vi "bbauv_acoustic.vi"() -> ()   [LabVIEW 2012]
doc: "This VI will initialize the FPGA VI and read a user-defined number of samples from a DMA FIFO. When the data acquisition is complete this VI will read status information from the FPGA VI.\n\nFollow these instructions to run the VI.\n\n1. Select your RIO device from the dropdown.\n2. Set the sample period, number of samples to acquire per channel, and DMA block read size. \n\nNote: the block read size should be set to balance load on the host processor and the update rate of the user interface. A small block read size will update the user interface more often but will result in a higher load on the host processor."
uses:
  <vilib>/userdefined/High Color/nirio_resource_hc.ctl
  <vilib>/FPGAPlugInAG/sbRIO-9612/niLvFpga_Open_sbRIO-9612.vi
  <vilib>/rvi/interface/common/dynamic/niFpgaDynamicAddResources.vi
  <vilib>/Utility/error.llb/Error Cluster From Error Code.vi
  <vilib>/FPGAPlugInAG/Dynamic/niLvFpga_Run_Dynamic.vi
  <vilib>/rvi/errors/niLvFpgaAdjustHostInterfaceError.vi
  <vilib>/RVI Host/nirviSupport.llb/nirviErrorClusterFromErrorCode.vi
  <vilib>/FPGAPlugInAG/Dynamic/niLvFpga_Close_Dynamic.vi
  <vilib>/express/express analysis/Spectral/Block/exnSpectralBlock spectral measurements peak poly.vi
  <vilib>/express/express analysis/Spectral/Block/exnSpectralBlock spectral measurements peak DDT.vi
  <vilib>/rvi/interface/nirviOpenFPGA/nirviOpenFPGA.xnode
  FPGA Bitfiles/bbauvFPGA_FPGATarget2_NI9223User-Contr_AXBjtBmtN8Y.lvbitx
  NI 9223 User-Controlled IO Sampling (FPGA).vi
  <vilib>/rvi/interface/nirviMethod/nirviMethod.xnode
  <vilib>/rvi/interface/nirviReadWriteControl/nirviReadWriteControl.xnode
  <vilib>/rvi/interface/nirviCloseFPGA/nirviCloseFPGA.xnode
  <vilib>/express/express analysis/Spectral/XNode/ExpressSpectralMeasurementsBlockNode.xnode
  <vilib>/rvi/errors/niLvFpgaMergeErrorWithErrorCode.vi
  <vilib>/rvi/interface/Simulation/niFpgaSimulationCallBeginRW.vi
  <vilib>/FPGAPlugInAG/Dynamic/niLvFpga_ReadFifo_Dynamic.vi
  <vilib>/rvi/interface/nirviMethod/StockFPGA_InlinedMethodWaitForSingleIRQ.vi
  <vilib>/FPGAPlugInAG/Dynamic/niLvFpga_WaitOnIrq_Dynamic.vi
  <vilib>/FPGAPlugInAG/Dynamic/niLvFpga_AcknowledgeIrq_Dynamic.vi
  NiFpgaLv.dll
  <vilib>/FPGAPlugInAG/Dynamic/niLvFpga_ConfigureFifo_Dynamic.vi
  <vilib>/FPGAPlugInAG/Dynamic/niLvFpga_StartFifo_Dynamic.vi
panel:
  out "Yaw Chart":dbl(graph)
  in  "Operating Mode":T1(ring)=enum."Analyze Real-time"
  in  "Filename":path=path "D:/Record Signal/sig 1.lvm"
  out "dt1":dbl
  out "dt2":dbl
  out "dt3":dbl
  out "Index 0":dbl
  out "Index 1":dbl
  out "Index 2":dbl
  out "Index 3":dbl
  out "ratio":dbl
  out "ratio 2":dbl
  out "ratio 3":dbl
  out "ratio 4":dbl
  out "amplitude":dbl
  out "amplitude 2":dbl
  out "amplitude 3":dbl
  out "amplitude 4":dbl
  out "ROS  Error":bool
  in  "Manual depth":dbl=4.3
  in  "Mode":T2(ring)=enum."Use Far Field"
  out "x":dbl format="%#_6f"
  out "y":dbl format="%#_6f"
  out "z":dbl
  out "yaw":dbl
  out "pitch":dbl
  out "Selected Index":i32
  in  "LPF Cut-Off":dbl=40000.0 caption="Lower Cut-Off"
  out "Ratio at Index (%)":dbl
  in  "Portion Duration":i32=200
  in  "peak min":dbl=0.1
  in  "Threshold":dbl=0.1
  out "Freq Domain":dynamicdata(graph)
  out "#element acquired":u32(graph)
  in  "Sampling Duration (us)":u32=2050000
  in  "RIO Device":T3="rio://192.168.0.150/RIO0"
  out "Timed Out":bool
  out "Sample Gated":bool
  out "Overwrite":bool
  in  "Acquisition Stop":bool
  out "Portion":dynamicdata(graph)
  out "Orignal Signal":dynamicdata(graph)
  # "Peak Finding"
  # "Triangulation Result"
  # "Operating Control"
  # "TDOA (us)"
  # "Signal Analysis Control"
  # "Signal Acquisition Control"
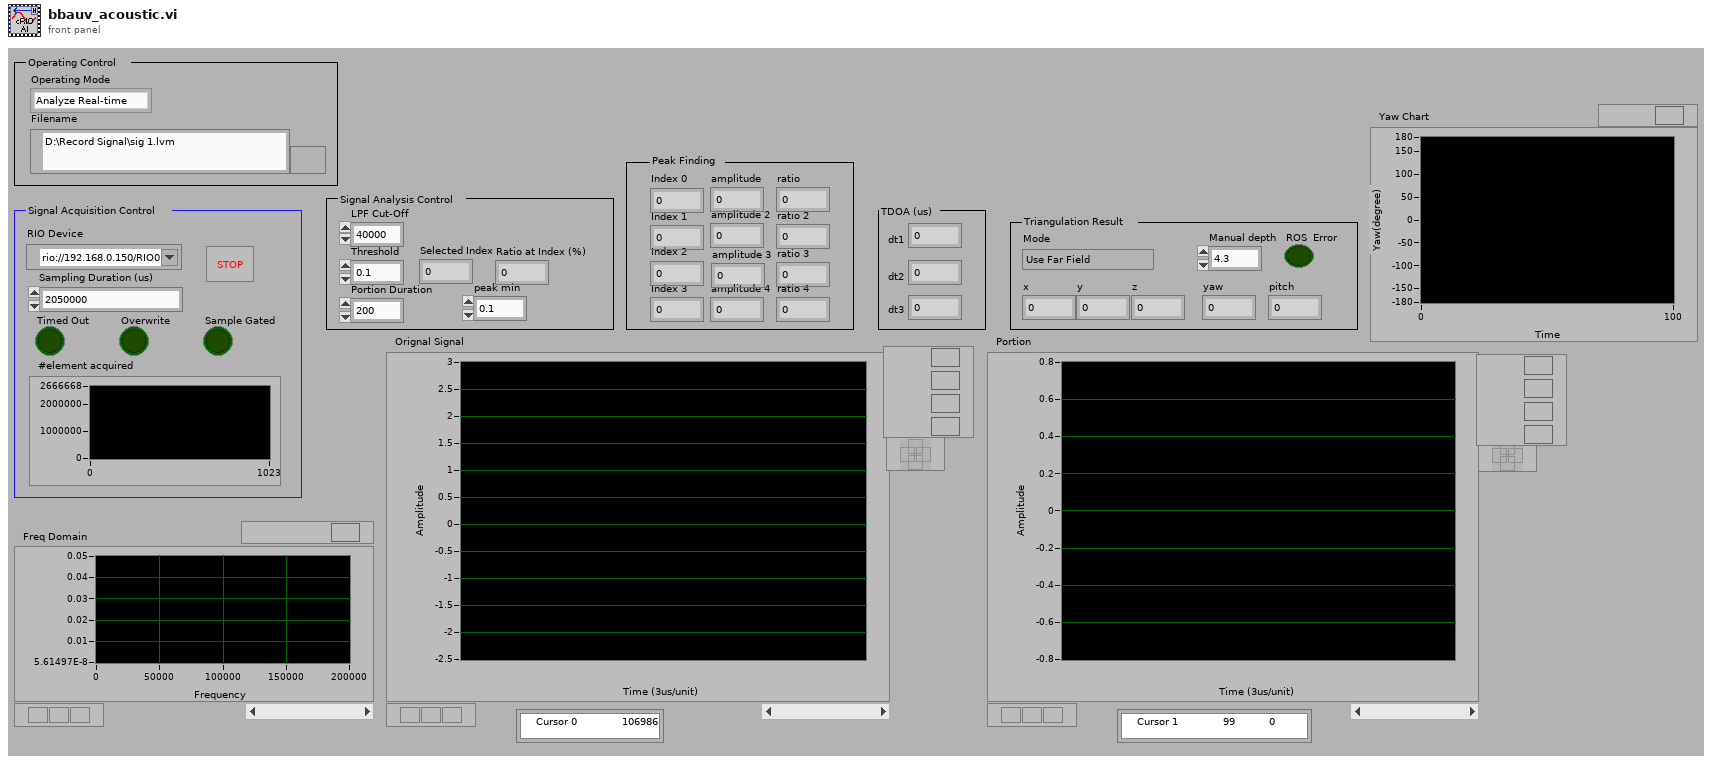
[diagram p1: front panel]
types:
  T1 = enum16{"Analyze From File", "Record Data", "Analyze Real-time"}
  T2 = enum16{"Use Near Field", "Use Far Field", "Send to ROS", "Far Field with 3 hydrophones"}
  T3 = typedef "nirio_resource_hc.ctl" = tag
  T4 = cluster{"averaging mode":u16, "weighting mode":u16, "number of averages":u32}
  T5 = cluster{"dB On (F)":bool, "unwrap phase (F)":bool, "convert to degree (F)":bool}
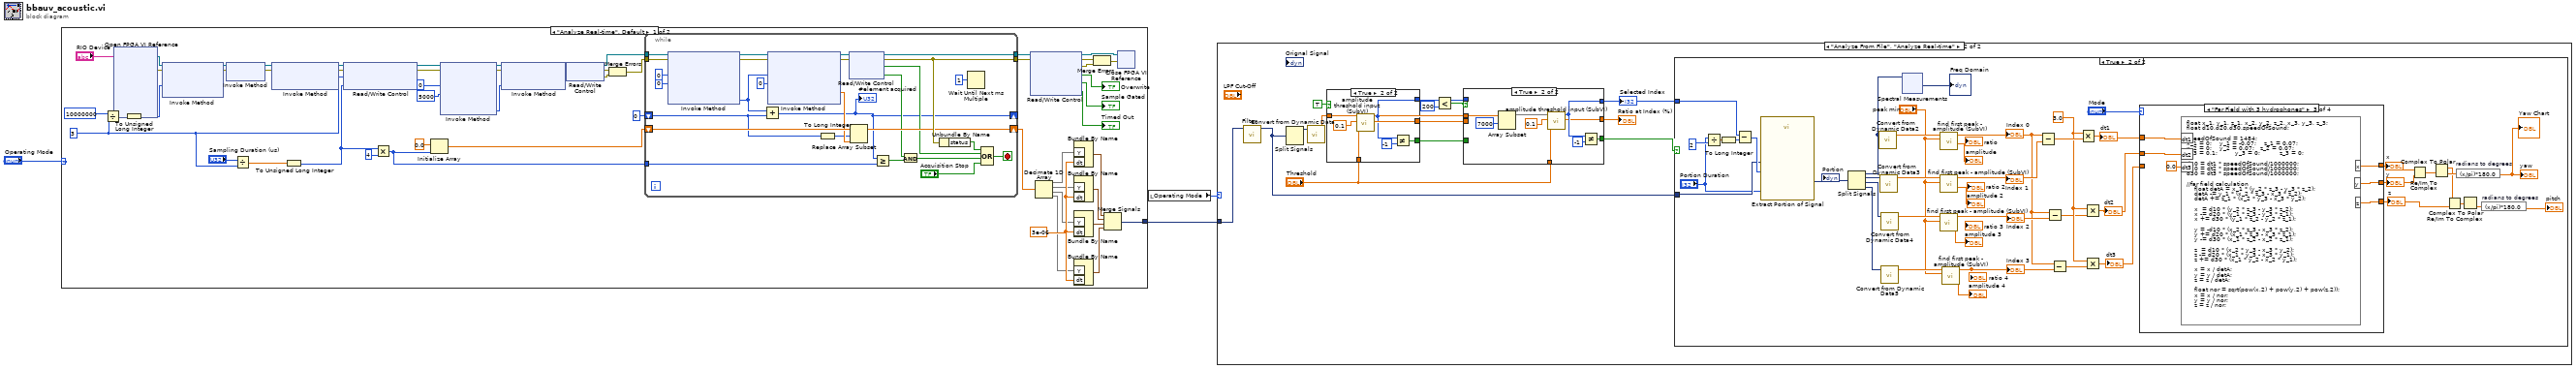
[diagram p0: block diagram]
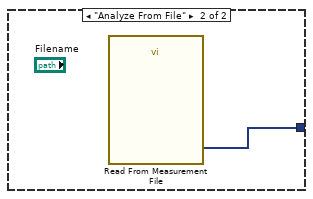
[diagram p2: hidden frame]
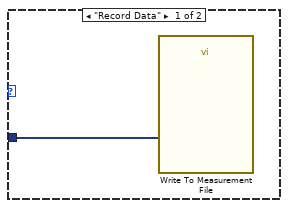
[diagram p3: hidden frame]
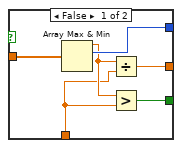
[diagram p5: hidden frame]
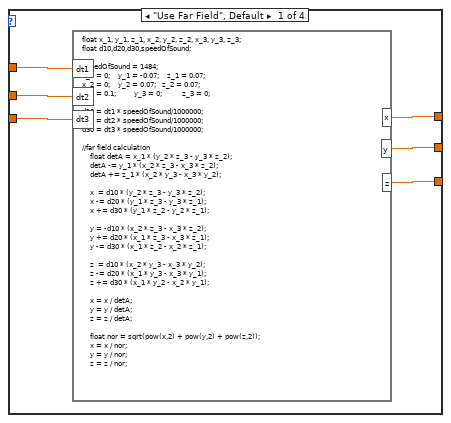
[diagram p7: hidden frame]
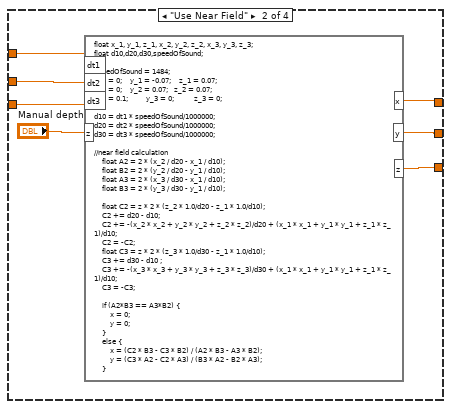
[diagram p8: hidden frame]
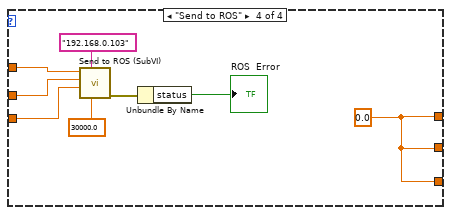
[diagram p9: hidden frame]
diagram:
  n1 = case shown="\"Analyze Real-time\", Default" "Operating Mode" {
    tunnel: [w8 w85] -> w3
    frame "Analyze Real-time", Default {
      w7 = u32 3 ("Sample Period (uSec)")
      w17 = 3e-06 ("dt")
      n2 = Divide(x=u32 10000000, y=w7) -> (x/y=w51:dbl)
      n3 = xnode "Open FPGA VI Reference"("resource name"="RIO Device") -> ("FPGA VI Reference Out"=w54:refnum<k20>, "error out"=w53:errorcluster)  [unwired: 1 in]
      n4 = To Unsigned Long Integer(number=w51) -> (unsigned 32bit integer=w52:u32)
      n5 = xnode "Invoke Method"("FPGA VI Reference In"=w54, "error in"=w53, "Requested Depth"=w52) -> ("FPGA VI Reference Out"=w56:refnum<k20>, "error out"=w55:errorcluster)  [unwired: 1 out]
      n6 = xnode "Invoke Method"("FPGA VI Reference In"=w56, "error in"=w55) -> ("FPGA VI Reference Out"=w45:refnum<k20>, "error out"=w44:errorcluster)
      n7 = Divide(x="Sampling Duration (us)", y=w7) -> (x/y=w5:dbl)
      n8 = xnode "Invoke Method"("FPGA VI Reference In"=w45, "error in"=w44) -> ("FPGA VI Reference Out"=w21:refnum<k20>, "error out"=w20:errorcluster)  [unwired: 1 in]
      n9 = To Unsigned Long Integer(number=w5) -> (unsigned 32bit integer=w4:u32)
      n10 = xnode "Read/Write Control"("FPGA VI Reference In"=w21, "error in"=w20, "Sample Period (uSec)"=w7, "Number of Samples"=w4) -> ("FPGA VI Reference Out"=w35:refnum<k20>, "error out"=w34:errorcluster)
      n11 = Multiply(x=w4, y=u32 4) -> (x*y=w48:u32)
      n12 = Initialize Array(sgl 0.0, w48) -> (w24:sgl[])
      n13 = xnode "Invoke Method"("FPGA VI Reference In"=w35, "error in"=w34, "IRQ Number(s)"=0, "Timeout (ms)"=5000) -> ("FPGA VI Reference Out"=w32:refnum<k20>, "error out"=w33:errorcluster, "IRQ(s) Asserted"=w29:i32)  [unwired: 1 out]
      n14 = xnode "Invoke Method"("FPGA VI Reference In"=w32, "error in"=w33, "IRQ Number(s)"=w29) -> ("FPGA VI Reference Out"=w31:refnum<k20>, "error out"=w30:errorcluster)
      n15 = xnode "Read/Write Control"("FPGA VI Reference In"=w31, "error in"=w30) -> ("FPGA VI Reference Out"=w23:refnum<k20>, "error out"=w37:errorcluster, "Error Out"=w36:errorcluster)
      n16 = Merge Errors(w37, w36) -> (w22:errorcluster)
      n17 = while {
        tunnel: w23 -> [w71]
        tunnel: w22 -> [w70]
        tunnel: [w79] -> w43
        tunnel: [w78] -> w42
        shift-right: [w58] -> _
        shift-left: u32 0 -> [w72]
        tunnel: w48 -> [w63]
        shift-right: [w74] -> w13
        shift-left: w24 -> [w80]
        stop <- w81 stop-if-true
        n18 = xnode "Invoke Method"("FPGA VI Reference In"=w71, "error in"=w70, "Number of Elements"=u32 0, "Timeout (ms)"=0) -> ("FPGA VI Reference Out"=w69:refnum<k20>, "error out"=w68:errorcluster, "Elements Remaining"=w59:u32)  [unwired: 1 out]
        n19 = Add(x=w59, y=w72) -> (x+y=w58:u32)
        "#element acquired" <- w58
        n20 = xnode "Invoke Method"("FPGA VI Reference In"=w69, "error in"=w68, "Number of Elements"=w59, "Timeout (ms)"=0) -> ("FPGA VI Reference Out"=w84:refnum<k20>, "error out"=w83:errorcluster, "Data"=w75:sgl[])  [unwired: 1 out]
        n21 = To Long Integer(number=w72) -> (32bit integer=w73:i32)
        n22 = xnode "Read/Write Control"("FPGA VI Reference In"=w84, "error in"=w83) -> ("FPGA VI Reference Out"=w79:refnum<k20>, "error out"=w78:errorcluster, "Error"=w60:bool, "Stopped"=w62:bool)
        n23 = Replace Array Subset(array=w80, new element=w75, index=w73) -> (w74:sgl[])
        n24 = Greater Or Equal?(x=w58, y=w63) -> (x >= y?=w64:bool)
        n25 = And(x=w62, y=w64) -> (x .and. y?=w61:bool)
        n26 = Unbundle By Name(w78) -> ("status"=w65:bool)
        n27 = Wait Until Next ms Multiple(millisecond multiple=u32 1) -> ()  [unwired: 1 out]
        n28 = Compound Arithmetic op=OR(w65, w60, w61, "Acquisition Stop") -> (w81:bool)
      }
      n29 = xnode "Read/Write Control"("FPGA VI Reference In"=w43, "error in"=w42) -> ("FPGA VI Reference Out"=w47:refnum<k20>, "error out"=w38:errorcluster, "Error Out"=w39:errorcluster, "Overwrite"=→"Overwrite":bool, "Sample Gated"=→"Sample Gated":bool, "Timed Out"=→"Timed Out":bool)
      n30 = Decimate 1D Array(w13) -> (w12:sgl[], w11:sgl[], w9:sgl[], w10:sgl[])
      n31 = Bundle By Name("Y"=w12, "dt"=w17) -> (w14:waveform(sgl))  [unwired: 1 in]
      n32 = Bundle By Name("Y"=w11, "dt"=w17) -> (w15:waveform(sgl))  [unwired: 1 in]
      n33 = Bundle By Name("Y"=w9, "dt"=w17) -> (w16:waveform(sgl))  [unwired: 1 in]
      n34 = Bundle By Name("Y"=w10, "dt"=w17) -> (w18:waveform(sgl))  [unwired: 1 in]
      n35 = Merge Errors(w38, w39) -> (w46:errorcluster)
      n36 = Merge Signals(w14, w15, w16, w18) -> (w8:dynamicdata)
      n37 = xnode "Close FPGA VI Reference"("FPGA VI Reference In"=w47, "error in"=w46) -> ()  [unwired: 1 out]
    }
    frame "Analyze From File" {
      n38 = call "Read From Measurement File"() -> ("Signals"=w85:dynamicdata)  [unwired: 6 in, 5 out]
    }
  }
  n39 = local read "Operating Mode"() -> (w2:T1)
  n40 = case shown="\"Analyze From File\", \"Analyze Real-time\"" w2 {
    tunnel: w3 -> [w86 w88]
    frame "Record Data" {
      n41 = call "Write To Measurement File"("Signals"=w86) -> ()  [unwired: 16 in, 3 out]
    }
    frame "Analyze From File", "Analyze Real-time" {
      n42 = call "Filter"("Signal"=w88) -> ("Filtered Signal"=w89:dynamicdata)  [unwired: 9 in, 1 out]
      n43 = Split Signals(w89) -> (w87:dynamicdata)  [unwired: 4 in, 3 out]
      n44 = call "Convert from Dynamic Data"("Dynamic Data Type"=w87) -> ("Array"=w95:dbl[])  [unwired: 3 in]
      n45 = case shown="True" TRUE {
        tunnel: w95 -> [w118 w125]
        tunnel: [w115 w122] -> w96
        tunnel: [w116 w121] -> w91
        tunnel: [w117 w120] -> w99
        tunnel: "Threshold" -> [w113 w119]
        frame False {
          n46 = Array Max & Min(array=w118) -> (max value=w114:dbl, max index (indices)=w116:i32)  [unwired: 2 out]
          n47 = Divide(x=w114, y=w113) -> (x/y=w115:dbl)
          n48 = Greater?(x=w114, y=w113) -> (0:w117:bool)
        }
        frame True {
          n49 = call "amplitude threshold input (SubVI).vi"("threshold"=w119, "%max amplitude"=0.1, "Array"=w125) -> ("actual ratio (%)"=w122:dbl, "Index"=w121:i32)  [unwired: 7 in]
          n50 = Not Equal?(x=w121, y=-1) -> (x != y?=w120:bool)
        }
      }
      n51 = Less?(x=w91, y=200) -> (x < y?=w97:bool)
      n52 = case shown="True" w97 {
        tunnel: w99 -> [w103 _]
        tunnel: w96 -> [w101 _]
        tunnel: w95 -> [_ w112]
        tunnel: "Threshold" -> [_ w107]
        tunnel: [w103 w106] -> w93
        tunnel: [w102 w105] -> w90
        tunnel: [w101 w104] -> w92
        tunnel: w91 -> [w102 _]
        frame False {
        }
        frame True {
          n53 = Array Subset(array=w112, index=7000) -> (w108:dbl[])  [unwired: 1 in]
          n54 = call "amplitude threshold input (SubVI).vi"("threshold"=w107, "%max amplitude"=0.1, "Array"=w108) -> ("actual ratio (%)"=w104:dbl, "Index"=w105:i32)  [unwired: 7 in]
          n55 = Not Equal?(x=w105, y=-1) -> (x != y?=w106:bool)
        }
      }
      "Ratio at Index (%)" <- w92
      "Selected Index" <- w90
      n56 = case shown="True" w93 {
        tunnel: w89 -> [_ w166]
        tunnel: w90 -> [_ w132]
        frame False {
        }
        frame True {
          w162 = 3.0 ("x")
          n57 = Divide(x="Portion Duration", y=2) -> (x/y=w136:dbl)
          n58 = To Long Integer(number=w136) -> (32bit integer=w135:i32)
          n59 = Subtract(x=w132, y=w135) -> (x-y=w169:i32)
          n60 = call "Extract Portion of Signal"("Samples"="Portion Duration", "Begin Sample"=w169, "Signals"=w166) -> ("Section"=w165:dynamicdata)  [unwired: 7 in, 1 out]
          "Portion" <- w165
          n61 = Split Signals(w165) -> (w126:dynamicdata, w168:dynamicdata, w167:dynamicdata, w164:dynamicdata)  [unwired: 4 in]
          n62 = call "Convert from Dynamic Data2"("Dynamic Data Type"=w126) -> ("Array"=w157:dbl[])  [unwired: 3 in]
          n63 = call "Convert from Dynamic Data3"("Dynamic Data Type"=w168) -> ("Array"=w156:dbl[])  [unwired: 3 in]
          n64 = call "Convert from Dynamic Data4"("Dynamic Data Type"=w167) -> ("Array"=w155:dbl[])  [unwired: 3 in]
          n65 = call "Convert from Dynamic Data5"("Dynamic Data Type"=w164) -> ("Array"=w154:dbl[])  [unwired: 3 in]
          n66 = xnode "Spectral Measurements"("Signals"=w126) -> ("FFT - (Peak)"=→"Freq Domain":dynamicdata)  [unwired: 1 in, 2 out]
          n67 = call "find first peak - amplitude (SubVI).vi"("min peak amplitude"="peak min", "Array"=w155) -> ("amplitude"=→"amplitude 3":dbl, "Index"=w152:dbl)  [unwired: 6 in, 1 out]
          "Index 2" <- w152
          n68 = call "find first peak - amplitude (SubVI).vi"("min peak amplitude"="peak min", "Array"=w157) -> ("amplitude"=→"amplitude":dbl, "Index"=w151:dbl)  [unwired: 6 in, 1 out]
          "Index 0" <- w151
          n69 = call "find first peak - amplitude (SubVI).vi"("min peak amplitude"="peak min", "Array"=w156) -> ("amplitude"=→"amplitude 2":dbl, "Index"=w153:dbl)  [unwired: 6 in, 1 out]
          "Index 1" <- w153
          n70 = call "find first peak - amplitude (SubVI).vi"("min peak amplitude"="peak min", "Array"=w154) -> ("amplitude"=→"amplitude 4":dbl, "Index"=w150:dbl)  [unwired: 6 in, 1 out]
          "Index 3" <- w150
          n71 = Subtract(x=w151, y=w153) -> (x-y=w163:dbl)
          n72 = Subtract(x=w151, y=w152) -> (x-y=w161:dbl)
          n73 = Subtract(x=w151, y=w150) -> (x-y=w160:dbl)
          n74 = Multiply(x=w162, y=w163) -> (x*y=w139:dbl)
          "dt1" <- w139
          n75 = Multiply(x=w162, y=w161) -> (x*y=w159:dbl)
          "dt2" <- w159
          n76 = Multiply(x=w162, y=w160) -> (x*y=w138:dbl)
          "dt3" <- w138
          n77 = case shown="\"Far Field with 3 hydrophones\"" "Mode" {
            tunnel: w139 -> [w185 w192 w198 w205]
            tunnel: w159 -> [w184 w191 w197 w204]
            tunnel: [w183 w190 w195 w202] -> w146
            tunnel: [w182 w189 w194 w202] -> w145
            tunnel: [w181 w188 w193 w202] -> w144
            tunnel: w138 -> [w180 w186 _ w201]
            frame "Use Far Field", Default {
              n78 = formula code="float x_1, y_1, z_1, x_2, y_2, z_2, x_3, y_3, z_3;\nfloat d10,d20,d30,speedOfSound;\n\nspeedOfSound = 1484;\nx_1 = 0;    y_1 = -0.07;    z_1 = 0.07;\nx_2 = 0;    y_2 = 0.07;   z_2 = 0.07;\nx_3 = 0.1;         y_3 = 0;          z_3 = 0;\n\nd10 = dt1 * speedOfSound/1000000;\nd20 = dt2 * speedOfSound/1000000;\nd30 = dt3 * speedOfSound/1000000;\n\n//far field calculation\n    float detA = x_1 * (y_2 * z_3 - y_3 * z_2);\n    detA -= y_1 * (x_2 * z_3 - x_3 * z_2);\n    detA += z_1 * (x_2 * y_3 - x_3 * y_2);\n\n    x  = d10 * (y_2 * z_3 - y_3 * z_2);\n    x -= d20 * (y_1 * z_3 - y_3 * z_1);\n    x += d30 * (y_1 * z_2 - y_2 * z_1);\n\n    y = -d10 * (x_2 * z_3 - x_3 * z_2);\n    y += d20 * (x_1 * z_3 - x_3 * z_1);\n    y -= d30 * (x_1 * z_2 - x_2 * z_1);\n\n    z  = d10 * (x_2 * y_3 - x_3 * y_2);\n    z -= d20 * (x_1 * y_3 - x_3 * y_1);\n    z += d30 * (x_1 * y_2 - x_2 * y_1);\n\n    x = x / detA;\n    y = y / detA;\n    z = z / detA;\n\n    float nor = sqrt(pow(x,2) + pow(y,2) + pow(z,2));\n    x = x / nor;\n    y = y / nor;\n    z = z / nor;"("dt1"=w185, "dt2"=w184, "dt3"=w180) -> ("x"=w183:dbl, "y"=w182:dbl, "z"=w181:dbl)
            }
            frame "Use Near Field" {
              n79 = formula code="float x_1, y_1, z_1, x_2, y_2, z_2, x_3, y_3, z_3;\nfloat d10,d20,d30,speedOfSound;\n\nspeedOfSound = 1484;\nx_1 = 0;    y_1 = -0.07;    z_1 = 0.07;\nx_2 = 0;    y_2 = 0.07;   z_2 = 0.07;\nx_3 = 0.1;         y_3 = 0;          z_3 = 0;\n\nd10 = dt1 * speedOfSound/1000000;\nd20 = dt2 * speedOfSound/1000000;\nd30 = dt3 * speedOfSound/1000000;\n\n//near field calculation\n    float A2 = 2 * (x_2 / d20 - x_1 / d10);\n    float B2 = 2 * (y_2 / d20 - y_1 / d10);\n    float A3 = 2 * (x_3 / d30 - x_1 / d10);\n    float B3 = 2 * (y_3 / d30 - y_1 / d10);\n    \n    float C2 = z * 2 * (z_2 * 1.0/d20 - z_1 * 1.0/d10);\n    C2 += d20 - d10;\n    C2 += -(x_2 * x_2 + y_2 * y_2 + z_2 * z_2)/d20 + (x_1 * x_1 + y_1 * y_1 + z_1 * z_1)/d10;\n    C2 = -C2;\n    float C3 = z * 2 * (z_3 * 1.0/d30 - z_1 * 1.0/d10);\n    C3 += d30 - d10 ;\n    C3 += -(x_3 * x_3 + y_3 * y_3 + z_3 * z_3)/d30 + (x_1 * x_1 + y_1 * y_1 + z_1 * z_1)/d10;\n    C3 = -C3;\n\n    if (A2*B3 == A3*B2) {\n        x = 0;\n        y = 0;\n    }\n    else {\n        x = (C2 * B3 - C3 * B2) / (A2 * B3 - A3 * B2);\n        y = (C3 * A2 - C2 * A3) / (B3 * A2 - B2 * A3);\n    }"("dt1"=w192, "dt2"=w191, "dt3"=w186, "z"="Manual depth") -> ("x"=w190:dbl, "y"=w189:dbl, "z"=w188:dbl)
            }
            frame "Far Field with 3 hydrophones" {
              n80 = formula code="float x_1, y_1, z_1, x_2, y_2, z_2, x_3, y_3, z_3;\nfloat d10,d20,d30,speedOfSound;\n\nspeedOfSound = 1484;\nx_1 = 0;    y_1 = -0.07;    z_1 = 0.07;\nx_2 = 0;    y_2 = 0.07;   z_2 = 0.07;\nx_3 = 0.1;         y_3 = 0;          z_3 = 0;\n\nd10 = dt1 * speedOfSound/1000000;\nd20 = dt2 * speedOfSound/1000000;\nd30 = dt3 * speedOfSound/1000000;\n\n//far field calculation\n    float detA = x_1 * (y_2 * z_3 - y_3 * z_2);\n    detA -= y_1 * (x_2 * z_3 - x_3 * z_2);\n    detA += z_1 * (x_2 * y_3 - x_3 * y_2);\n\n    x  = d10 * (y_2 * z_3 - y_3 * z_2);\n    x -= d20 * (y_1 * z_3 - y_3 * z_1);\n    x += d30 * (y_1 * z_2 - y_2 * z_1);\n\n    y = -d10 * (x_2 * z_3 - x_3 * z_2);\n    y += d20 * (x_1 * z_3 - x_3 * z_1);\n    y -= d30 * (x_1 * z_2 - x_2 * z_1);\n\n    z  = d10 * (x_2 * y_3 - x_3 * y_2);\n    z -= d20 * (x_1 * y_3 - x_3 * y_1);\n    z += d30 * (x_1 * y_2 - x_2 * y_1);\n\n    x = x / detA;\n    y = y / detA;\n    z = z / detA;\n\n    float nor = sqrt(pow(x,2) + pow(y,2) + pow(z,2));\n    x = x / nor;\n    y = y / nor;\n    z = z / nor;"("dt1"=w198, "dt2"=w197, "dt3"=0.0 ("input variable")) -> ("x"=w195:dbl, "y"=w194:dbl, "z"=w193:dbl)
            }
            frame "Send to ROS" {
              w202 = 0.0 ("x")
              n81 = call "Send to ROS (SubVI).vi"("frequency"=30000.0, "ROS IP"="192.168.0.103", "dt 3"=w201, "dt2"=w204, "dt 1"=w205) -> ("error out"=w200:errorcluster)  [unwired: 6 in]
              n82 = Unbundle By Name(w200) -> ("status"=→"ROS  Error":bool)
            }
          }
          "x" <- w146
          "y" <- w145
          "z" <- w144
          n83 = Re/Im To Complex(1:w145, 2:w146) -> (0:w148:cdb)
          n84 = Complex To Polar(r * e^(i*theta)=w148) -> (r=w143:dbl, theta=w147:dbl)
          n85 = Re/Im To Complex(1:w144, 2:w143) -> (0:w142:cdb)
          n86 = expression code="(x/pi)*180.0" "radians to degrees"(w147) -> (→"yaw" →"Yaw Chart":dbl)
          n87 = Complex To Polar(r * e^(i*theta)=w142) -> (theta=w140:dbl)  [unwired: 1 out]
          n88 = expression code="(x/pi)*180.0" "radians to degrees"(w140) -> (→"pitch":dbl)
        }
      }
    }
  }
